vi "[RT] eHS Main.vi"() -> ()   [LabVIEW 2017]
uses:
  <vilib>/userdefined/High Color/nirio_resource_hc.ctl
  <vilib>/NI/cRIO Wfm/ChannelConfig.ctl
  <vilib>/OPAL-RT/Utilities Toolkit/Mapping/Input Mapping/Common/Controls/Input Mapping Parameters.ctl
  <vilib>/OPAL-RT/Utilities Toolkit/Mapping/Input Mapping/Common/Controls/Input Source Types.ctl
  <vilib>/OPAL-RT/Utilities Toolkit/Mapping/Switch Mapping/Common/Controls/Switch Mapping Parameters.ctl
  <vilib>/OPAL-RT/Utilities Toolkit/Mapping/Switch Mapping/Common/Controls/Switch Source Types.ctl
  <vilib>/OPAL-RT/Analog I-O Mapping & Conditioning Toolkit/AOMC/Common/Public/Controls/AOMC Configuration Parameters.ctl
  <vilib>/OPAL-RT/Analog I-O Mapping & Conditioning Toolkit/AOMC/Common/Public/Controls/AO Mapping Parameters.ctl
  <vilib>/OPAL-RT/Analog I-O Mapping & Conditioning Toolkit/AOMC/Common/Public/Controls/Source Type.ctl
  <vilib>/OPAL-RT/Analog I-O Mapping & Conditioning Toolkit/AOMC/Common/Public/Controls/AO Conditioning Parameters.ctl
  <vilib>/OPAL-RT/eHS Toolkit/eHS Host/Controls/eHS Core Index.ctl
  <vilib>/OPAL-RT/FPGA Signal Generation Toolkit/Sinewave Generation/Host/Public/Controls/Phase Offset Mode.ctl
  <vilib>/OPAL-RT/FPGA Signal Generation Toolkit/Sinewave Generation/Host/Public/Controls/Sinewave FPGA Clock Rate.ctl
  <vilib>/OPAL-RT/FPGA Signal Generation Toolkit/Sinewave Generation/Host/Public/Controls/Sinewave RT Configuration Parameters.ctl
  <vilib>/OPAL-RT/FPGA Signal Generation Toolkit/Sinewave Generation/Host/Public/Controls/Sinewave Generator Action.ctl
  <vilib>/OPAL-RT/eHS Toolkit/eHS Host/SubVIs/eHS Core/eHSx64 Initialize Solver Core.vi
  <vilib>/OPAL-RT/Analog I-O Mapping & Conditioning Toolkit/AOMC/Host/Private/Pack & Send AOMC Configuration Setting.vi
  <vilib>/Utility/error.llb/Error Cluster From Error Code.vi
  <vilib>/rvi/errors/niLvFpgaAdjustHostInterfaceError.vi
  <vilib>/NI/cRIO Wfm/AcqRead(Wfm).vi
  <vilib>/FPGAPlugInAG/Dynamic/niLvFpga_Abort_Dynamic.vi
  <vilib>/FPGAPlugInAG/Dynamic/niLvFpga_Close_Dynamic.vi
  <vilib>/rvi/interface/nirviReadWriteControl/nirviReadWriteControl.xnode
  Controls/eHS FPGA Ref.ctl
  <vilib>/rvi/interface/nirviMethod/nirviMethod.xnode
  <vilib>/rvi/interface/nirviCloseFPGA/nirviCloseFPGA.xnode
  <vilib>/NI/cRIO Wfm/cRIO Wfm.lvlib
  <vilib>/OPAL-RT/eHS Toolkit/eHS Host/eHS - Host.lvlib
  <vilib>/OPAL-RT/Analog I-O Mapping & Conditioning Toolkit/AOMC/Host/AO Mapping & Conditioning - Host.lvlib
  <vilib>/OPAL-RT/FPGA Signal Generation Toolkit/Sinewave Generation/Host/Sinewave Generation - Host.lvlib
  <vilib>/rvi/interface/Simulation/niFpgaSimulationCallBeginRW.vi
  NiFpgaLv.dll
  <vilib>/OPAL-RT/Utilities Toolkit/Mapping/Input Mapping/Common/Input Mapping - Common.lvlib
  <vilib>/OPAL-RT/Utilities Toolkit/Mapping/Switch Mapping/Common/Switch Mapping - Common.lvlib
  <vilib>/OPAL-RT/Analog I-O Mapping & Conditioning Toolkit/AOMC/Common/AO Mapping & Conditioning - Common.lvlib
panel:
  in  "STOP":bool
  in  "eHS+PMSM Tab":T1(tab)=enum."Control & Monitor"
  in  "Resource name":T2="RIO0" caption="RIO Device"
  in  "Waveform Channel Info":T3=[{"Channel Name"="U01", "Sensitivity mV_EU"=1000.0, "EU"="V", "dB Ref EU"=1.0}, {"Channel Name"="U02", "Sensitivity mV_EU"=1000.0, "EU"="V", "dB Ref EU"=1.0}, {"Channel Name"="U03", "Sensitivity mV_EU"=1000.0, "EU"="V", "dB Ref EU"=1.0}, {"Channel Name"="U04", "Sensitivity mV_EU"=1000.0, "EU"="V", "dB Ref EU"=1.0}, {"Channel Name"="U05", "Sensitivity mV_EU"=1000.0, "EU"="V", "dB Ref EU"=1.0}, {"Channel Name"="U06", "Sensitivity mV_EU"=1000.0, "EU"="V", "dB Ref EU"=1.0}, {"Channel Name"="U07", "Sensitivity mV_EU"=1000.0, "EU"="V", "dB Ref EU"=1.0}, {"Channel Name"="U08", "Sensitivity mV_EU"=1000.0, "EU"="V", "dB Ref EU"=1.0}, {"Channel Name"="U09", "Sensitivity mV_EU"=1000.0, "EU"="V", "dB Ref EU"=1.0}, {"Channel Name"="U10", "Sensitivity mV_EU"=1000.0, "EU"="V", "dB Ref EU"=1.0}, {"Channel Name"="U11", "Sensitivity mV_EU"=1000.0, "EU"="V", "dB Ref EU"=1.0}, {"Channel Name"="U12", "Sensitivity mV_EU"=1000.0, "EU"="V", "dB Ref EU"=1.0}, {"Channel Name"="U13", "Sensitivity mV_EU"=1000.0, "EU"="V", "dB Ref EU"=1.0}, {"Channel Name"="U14", "Sensitivity mV_EU"=1000.0, "EU"="V", "dB Ref EU"=1.0}, {"Channel Name"="U15", "Sensitivity mV_EU"=1000.0, "EU"="V", "dB Ref EU"=1.0}, {"Channel Name"="U16", "Sensitivity mV_EU"=1000.0, "EU"="V", "dB Ref EU"=1.0}, {"Channel Name"="U17", "Sensitivity mV_EU"=1000.0, "EU"="V", "dB Ref EU"=1.0}, {"Channel Name"="U18", "Sensitivity mV_EU"=1000.0, "EU"="V", "dB Ref EU"=1.0}, {"Channel Name"="U19", "Sensitivity mV_EU"=1000.0, "EU"="V", "dB Ref EU"=1.0}, {"Channel Name"="U20", "Sensitivity mV_EU"=1000.0, "EU"="V", "dB Ref EU"=1.0}, {"Channel Name"="U21", "Sensitivity mV_EU"=1000.0, "EU"="V", "dB Ref EU"=1.0}, {"Channel Name"="U22", "Sensitivity mV_EU"=1000.0, "EU"="V", "dB Ref EU"=1.0}, {"Channel Name"="U23", "Sensitivity mV_EU"=1000.0, "EU"="V", "dB Ref EU"=1.0}, {"Channel Name"="U24", "Sensitivity mV_EU"=1000.0, "EU"="V", "dB Ref EU"=1.0}, {"Channel Name"="U25", "Sensitivity mV_EU"=1000.0, "EU"="V", "dB Ref EU"=1.0}, {"Channel Name"="U26", "Sensitivity mV_EU"=1000.0, "EU"="V", "dB Ref EU"=1.0}, {"Channel Name"="U27", "Sensitivity mV_EU"=1000.0, "EU"="V", "dB Ref EU"=1.0}, {"Channel Name"="U28", "Sensitivity mV_EU"=1000.0, "EU"="V", "dB Ref EU"=1.0}, {"Channel Name"="U29", "Sensitivity mV_EU"=1000.0, "EU"="V", "dB Ref EU"=1.0}, {"Channel Name"="U30", "Sensitivity mV_EU"=1000.0, "EU"="V", "dB Ref EU"=1.0}, {"Channel Name"="U31", "Sensitivity mV_EU"=1000.0, "EU"="V", "dB Ref EU"=1.0}, {"Channel Name"="U32", "Sensitivity mV_EU"=1000.0, "EU"="V", "dB Ref EU"=1.0}] {"dB Ref EU" format="%#.2p"; "Sensitivity mV_EU" format="%.2f"}
  in  "Waveform Buffer Size":i32=100000
  in  "Waveform Sample Rate":u32=88888
  in  "eHS Input Mapping Keys":T4[](array[typedef])=[{"Source Index"=0, "Input Source Types"=enum."Group B"}, {"Source Index"=1, "Input Source Types"=enum."Group B"}, {"Source Index"=2, "Input Source Types"=enum."Group B"}, {"Source Index"=3, "Input Source Types"=enum."Group B"}, {"Source Index"=4, "Input Source Types"=enum."Group B"}, {"Source Index"=5, "Input Source Types"=enum."Group B"}, {"Source Index"=0, "Input Source Types"=enum."Group A"}]
  in  "eHS Switch Mapping Keys":T6[](array[typedef])=[{"Switch Source Types"=enum."Group D", "Source Index"=0, "Invert?"=FALSE}, {"Switch Source Types"=enum."Group D", "Source Index"=1, "Invert?"=FALSE}, {"Switch Source Types"=enum."Group D", "Source Index"=2, "Invert?"=FALSE}, {"Switch Source Types"=enum."Group D", "Source Index"=3, "Invert?"=FALSE}, {"Switch Source Types"=enum."Group D", "Source Index"=4, "Invert?"=FALSE}, {"Switch Source Types"=enum."Group D", "Source Index"=5, "Invert?"=FALSE}, {"Switch Source Types"=enum."Group D", "Source Index"=6, "Invert?"=FALSE}, {"Switch Source Types"=enum."Group D", "Source Index"=7, "Invert?"=FALSE}, {"Switch Source Types"=enum."Group D", "Source Index"=8, "Invert?"=FALSE}, {"Switch Source Types"=enum."Group D", "Source Index"=9, "Invert?"=FALSE}, {"Switch Source Types"=enum."Group D", "Source Index"=10, "Invert?"=TRUE}, {"Switch Source Types"=enum."Group D", "Source Index"=11, "Invert?"=FALSE}]
  in  "AOMC Configuration Parameters":T8[](array[typedef])=[{"AO Mapping Parameters"={"AO Channel Index"=0, "Source"=enum."Group A", "Source Index"=8}, "AO Conditioning Parameters"={"Scaling Factor"=0.5, "Offset Factor"=0.0, "Minumum Saturation"=-10.0, "Maximum Saturation"=10.0}}, {"AO Mapping Parameters"={"AO Channel Index"=1, "Source"=enum."Group A", "Source Index"=9}, "AO Conditioning Parameters"={"Scaling Factor"=0.5, "Offset Factor"=0.0, "Minumum Saturation"=-10.0, "Maximum Saturation"=10.0}}, {"AO Mapping Parameters"={"AO Channel Index"=2, "Source"=enum."Not Connected", "Source Index"=0}, "AO Conditioning Parameters"={"Scaling Factor"=0.0, "Offset Factor"=0.0, "Minumum Saturation"=-10.0, "Maximum Saturation"=10.0}}, {"AO Mapping Parameters"={"AO Channel Index"=3, "Source"=enum."Not Connected", "Source Index"=0}, "AO Conditioning Parameters"={"Scaling Factor"=0.0, "Offset Factor"=0.0, "Minumum Saturation"=-10.0, "Maximum Saturation"=10.0}}, {"AO Mapping Parameters"={"AO Channel Index"=4, "Source"=enum."Group A", "Source Index"=6}, "AO Conditioning Parameters"={"Scaling Factor"=0.014793, "Offset Factor"=0.0, "Minumum Saturation"=-10.0, "Maximum Saturation"=10.0}}, {"AO Mapping Parameters"={"AO Channel Index"=5, "Source"=enum."Not Connected", "Source Index"=0}, "AO Conditioning Parameters"={"Scaling Factor"=0.0, "Offset Factor"=0.0, "Minumum Saturation"=0.0, "Maximum Saturation"=0.0}}, {"AO Mapping Parameters"={"AO Channel Index"=6, "Source"=enum."Not Connected", "Source Index"=0}, "AO Conditioning Parameters"={"Scaling Factor"=0.0, "Offset Factor"=0.0, "Minumum Saturation"=0.0, "Maximum Saturation"=0.0}}, {"AO Mapping Parameters"={"AO Channel Index"=7, "Source"=enum."Not Connected", "Source Index"=0}, "AO Conditioning Parameters"={"Scaling Factor"=0.0, "Offset Factor"=0.0, "Minumum Saturation"=0.0, "Maximum Saturation"=0.0}}, {"AO Mapping Parameters"={"AO Channel Index"=8, "Source"=enum."Group A", "Source Index"=3}, "AO Conditioning Parameters"={"Scaling Factor"=0.5, "Offset Factor"=0.0, "Minumum Saturation"=-10.0, "Maximum Saturation"=10.0}}, {"AO Mapping Parameters"={"AO Channel Index"=9, "Source"=enum."Group A", "Source Index"=4}, "AO Conditioning Parameters"={"Scaling Factor"=0.5, "Offset Factor"=0.0, "Minumum Saturation"=-10.0, "Maximum Saturation"=10.0}}, {"AO Mapping Parameters"={"AO Channel Index"=10, "Source"=enum."Group A", "Source Index"=5}, "AO Conditioning Parameters"={"Scaling Factor"=0.5, "Offset Factor"=0.0, "Minumum Saturation"=-10.0, "Maximum Saturation"=10.0}}, {"AO Mapping Parameters"={"AO Channel Index"=11, "Source"=enum."Group A", "Source Index"=7}, "AO Conditioning Parameters"={"Scaling Factor"=0.1, "Offset Factor"=0.0, "Minumum Saturation"=-10.0, "Maximum Saturation"=10.0}}, {"AO Mapping Parameters"={"AO Channel Index"=12, "Source"=enum."Group A", "Source Index"=0}, "AO Conditioning Parameters"={"Scaling Factor"=0.04714, "Offset Factor"=0.0, "Minumum Saturation"=-10.0, "Maximum Saturation"=10.0}}, {"AO Mapping Parameters"={"AO Channel Index"=13, "Source"=enum."Group A", "Source Index"=1}, "AO Conditioning Parameters"={"Scaling Factor"=0.04714, "Offset Factor"=0.0, "Minumum Saturation"=-10.0, "Maximum Saturation"=10.0}}, {"AO Mapping Parameters"={"AO Channel Index"=14, "Source"=enum."Group A", "Source Index"=2}, "AO Conditioning Parameters"={"Scaling Factor"=0.04714, "Offset Factor"=0.0, "Minumum Saturation"=-10.0, "Maximum Saturation"=10.0}}, {"AO Mapping Parameters"={"AO Channel Index"=15, "Source"=enum."Group A", "Source Index"=10}, "AO Conditioning Parameters"={"Scaling Factor"=0.014793, "Offset Factor"=0.0, "Minumum Saturation"=-10.0, "Maximum Saturation"=10.0}}]
  out "eHS Outputs":waveform(sgl)[](graph)=[{"t0"=timestamp(3605532672.448228 s since 1904-01-01), "dt"=1.1249999999999999e-05, "Y"=array[10000 elements], "attributes"=variant("NI_ChannelName"=variant(string "U04"), "NI_UnitDescription"=variant(string "V"), "NI_dBReference"=variant(dbl 1.0))}, {"t0"=timestamp(3605532672.448228 s since 1904-01-01), "dt"=1.1249999999999999e-05, "Y"=array[10000 elements], "attributes"=variant("NI_ChannelName"=variant(string "U05"), "NI_UnitDescription"=variant(string "V"), "NI_dBReference"=variant(dbl 1.0))}, {"t0"=timestamp(3605532672.448228 s since 1904-01-01), "dt"=1.1249999999999999e-05, "Y"=array[10000 elements], "attributes"=variant("NI_ChannelName"=variant(string "U06"), "NI_UnitDescription"=variant(string "V"), "NI_dBReference"=variant(dbl 1.0))}]
  in  "eHS Constant Inputs":sgl[](array[numeric])=[12.6, 0.0, 0.0, 0.0, 0.0, 0.0, 0.0, 0.0, 0.0, 0.0, 0.0, 0.0, 0.0, 0.0, 0.0, 0.0, 0.0, 0.0, 0.0, 0.0, 0.0, 0.0, 0.0, 0.0, 0.0, 0.0, 0.0, 0.0, 0.0, 0.0, 0.0, 0.0]
  in  "eHS SW Constants":bool[](array[boolean])=[FALSE, FALSE, FALSE, FALSE, FALSE, FALSE, FALSE, FALSE, FALSE, FALSE, FALSE, FALSE, FALSE, FALSE, FALSE, FALSE, FALSE, FALSE, FALSE, FALSE, FALSE, FALSE, FALSE, FALSE, FALSE, FALSE, FALSE, FALSE, FALSE, FALSE, FALSE, FALSE, FALSE, FALSE, FALSE, FALSE, FALSE, FALSE, FALSE, FALSE, FALSE, FALSE, FALSE, FALSE, FALSE, FALSE, FALSE, FALSE, FALSE, FALSE, FALSE, FALSE, FALSE, FALSE, FALSE, FALSE, FALSE, FALSE, FALSE, FALSE, FALSE, FALSE, FALSE, FALSE, FALSE, FALSE, FALSE, FALSE, FALSE, FALSE, FALSE, FALSE]
  in  "Waveform Selection":T12={"Boolean"=FALSE, "Boolean 2"=FALSE, "Boolean 3"=FALSE, "Boolean 4"=TRUE, "Boolean 5"=TRUE, "Boolean 6"=TRUE, "Boolean 7"=FALSE, "Boolean 8"=FALSE, "Boolean 9"=FALSE, "Boolean 10"=FALSE, "Boolean 11"=FALSE, "Boolean 12"=FALSE, "Boolean 13"=FALSE, "Boolean 14"=FALSE, "Boolean 15"=FALSE, "Boolean 16"=FALSE, "Boolean 17"=FALSE, "Boolean 18"=FALSE, "Boolean 19"=FALSE, "Boolean 20"=FALSE, "Boolean 21"=FALSE, "Boolean 22"=FALSE, "Boolean 23"=FALSE, "Boolean 24"=FALSE, "Boolean 25"=FALSE, "Boolean 26"=FALSE, "Boolean 27"=FALSE, "Boolean 28"=FALSE, "Boolean 29"=FALSE, "Boolean 30"=FALSE, "Boolean 31"=FALSE, "Boolean 32"=FALSE}
  out "Mapped & Conditioned Data_Debug":fxp<+/-,20,5>[](array[numeric])=[10.0, 10.0, 0.0, 0.0, 3.26995849609375, 0.0, 0.0, 0.0, 10.0, -8.520599365234375, 10.0, 3.556671142578125, 7.373077392578125, -3.07159423828125, -5.40924072265625, 3.2708740234375, 0.0, 0.0, 0.0, 0.0, 0.0, 0.0, 0.0, 0.0, 0.0, 0.0, 0.0, 0.0, 0.0, 0.0, 0.0, 0.0] format="%.17g"
  out "Conditioned AI Data_Debug":sgl[](array[numeric])
  # "Hardware Setup"
  # "RIO Waveform Settings"
  # "eHS U #"
  # "eHS SW #"
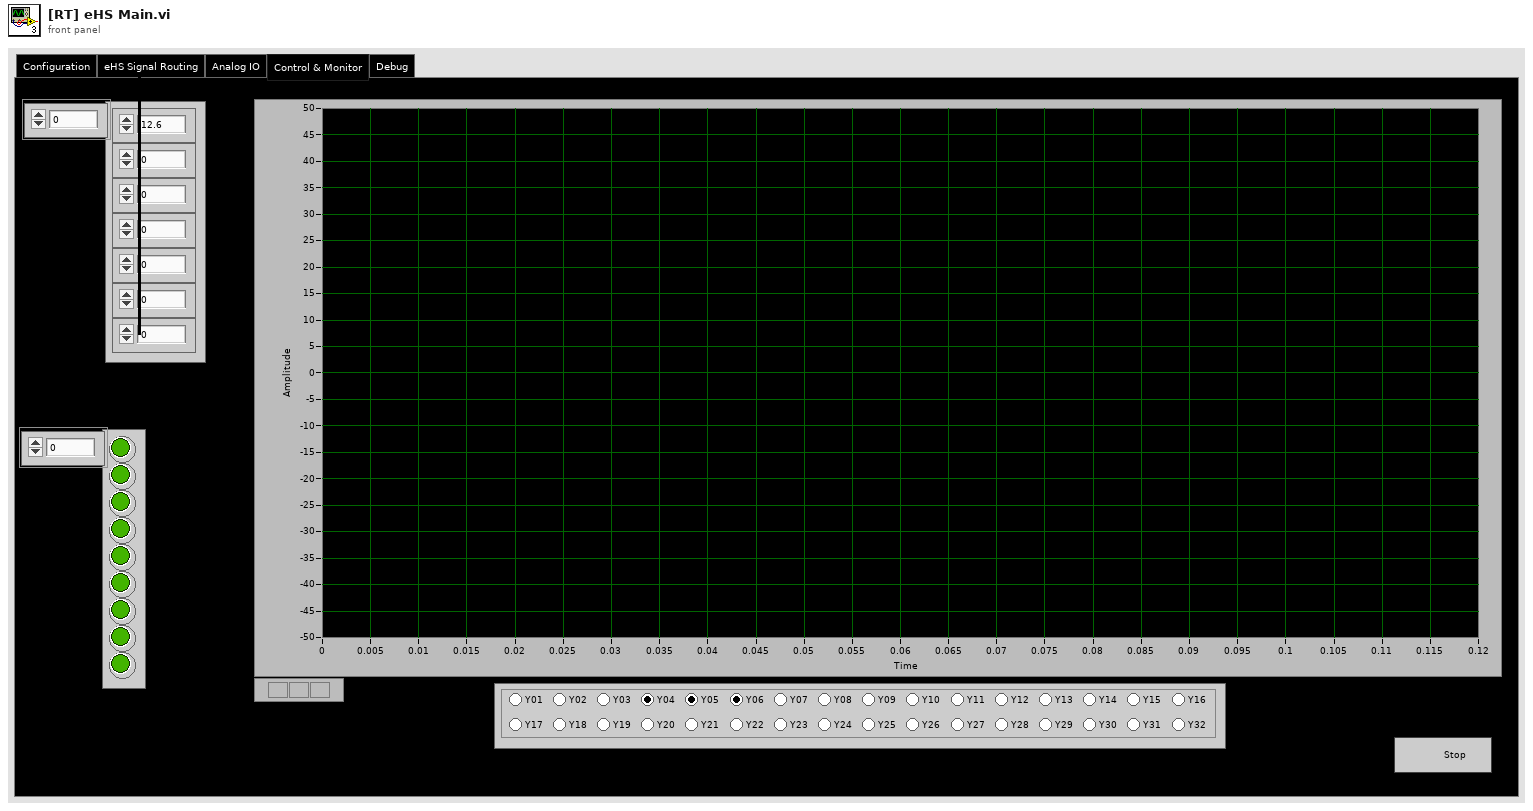
[diagram p1: front panel]
types:
  T1 = enum32{"Configuration", "eHS Signal Routing", "Analog IO", "Control & Monitor", "Debug"}
  T2 = typedef "nirio_resource_hc.ctl" = tag
  T3 = typedef "cRIO Wfm.lvlib/ChannelConfig.ctl" = cluster{"Channel Name":string, "Sensitivity mV_EU":dbl, "EU":string, "dB Ref EU":dbl}[]
  T4 = typedef "Input Mapping - Common.lvlib/Input Mapping Parameters.ctl" = cluster{"Source Index":u8, "Input Source Types":T5}
  T5 = typedef "Input Mapping - Common.lvlib/Input Source Types.ctl" = enum16{"Not Connected", "Group A", "Group B", "Group C", "Group D"}
  T6 = typedef "Switch Mapping - Common.lvlib/Switch Mapping Parameters.ctl" = cluster{"Switch Source Types":T7, "Source Index":u8, "Invert?":bool}
  T7 = typedef "Switch Mapping - Common.lvlib/Switch Source Types.ctl" = enum16{"Not Connected", "Group A", "Group B", "Group C", "Group D", "Group E"}
  T8 = typedef "AO Mapping & Conditioning - Common.lvlib/AOMC Configuration Parameters.ctl" = cluster{"AO Mapping Parameters":T9, "AO Conditioning Parameters":T11}
  T9 = typedef "AO Mapping & Conditioning - Common.lvlib/AO Mapping Parameters.ctl" = cluster{"AO Channel Index":u8, "Source":T10, "Source Index":u8}
  T10 = typedef "AO Mapping & Conditioning - Common.lvlib/Source Type.ctl" = enum16{"Not Connected", "Group A", "Group B"}
  T11 = typedef "AO Mapping & Conditioning - Common.lvlib/AO Conditioning Parameters.ctl" = cluster{"Scaling Factor":sgl, "Offset Factor":sgl, "Minumum Saturation":sgl, "Maximum Saturation":sgl}
  T12 = cluster{"Boolean":bool, "Boolean 2":bool, "Boolean 3":bool, "Boolean 4":bool, "Boolean 5":bool, "Boolean 6":bool, "Boolean 7":bool, "Boolean 8":bool, "Boolean 9":bool, "Boolean 10":bool, "Boolean 11":bool, "Boolean 12":bool, "Boolean 13":bool, "Boolean 14":bool, "Boolean 15":bool, "Boolean 16":bool, "Boolean 17":bool, "Boolean 18":bool, "Boolean 19":bool, "Boolean 20":bool, "Boolean 21":bool, "Boolean 22":bool, "Boolean 23":bool, "Boolean 24":bool, "Boolean 25":bool, "Boolean 26":bool, "Boolean 27":bool, "Boolean 28":bool, "Boolean 29":bool, "Boolean 30":bool, "Boolean 31":bool, "Boolean 32":bool}
  T13 = typedef "Sinewave Generation - Host.lvlib/Sinewave Generator Action.ctl" = enum16{"Do Nothing", "Stop", "Re-Start"}
  T14 = typedef "Sinewave Generation - Host.lvlib/Sinewave RT Configuration Parameters.ctl" = cluster{"Frequency Engine Index":u8, "Phase Offset (Deg\\Rad)":dbl, "Amplitude":dbl, "Offset":dbl}
  T15 = typedef "Sinewave Generation - Host.lvlib/Sinewave FPGA Clock Rate.ctl" = enum16{"50MHz", "100MHz"}
  T16 = typedef "Sinewave Generation - Host.lvlib/Phase Offset Mode.ctl" = enum16{"Degrees", "Radians"}
  T17 = typedef "OPAL-RT eHS.lvlib/eHS - Host.lvlib/eHS Core Index.ctl" = enum16{"Core 1", "Core 2", "Core 3", "Core 4", "Core 5", "Core 6", "Core 7", "Core 8", "Core 9", "Core 10"}
  T18 = typedef "eHS FPGA Ref.ctl" = refnum<k20>
  T19 = typedef "cRIO Wfm.lvlib/SamplingInfo.ctl" = cluster{"Number of Channels":i32, "Actual Samp Rate":dbl, "Chan Name Array":string[], "EU Chan Array":string[], "dB Ref Chan Array":dbl[]}
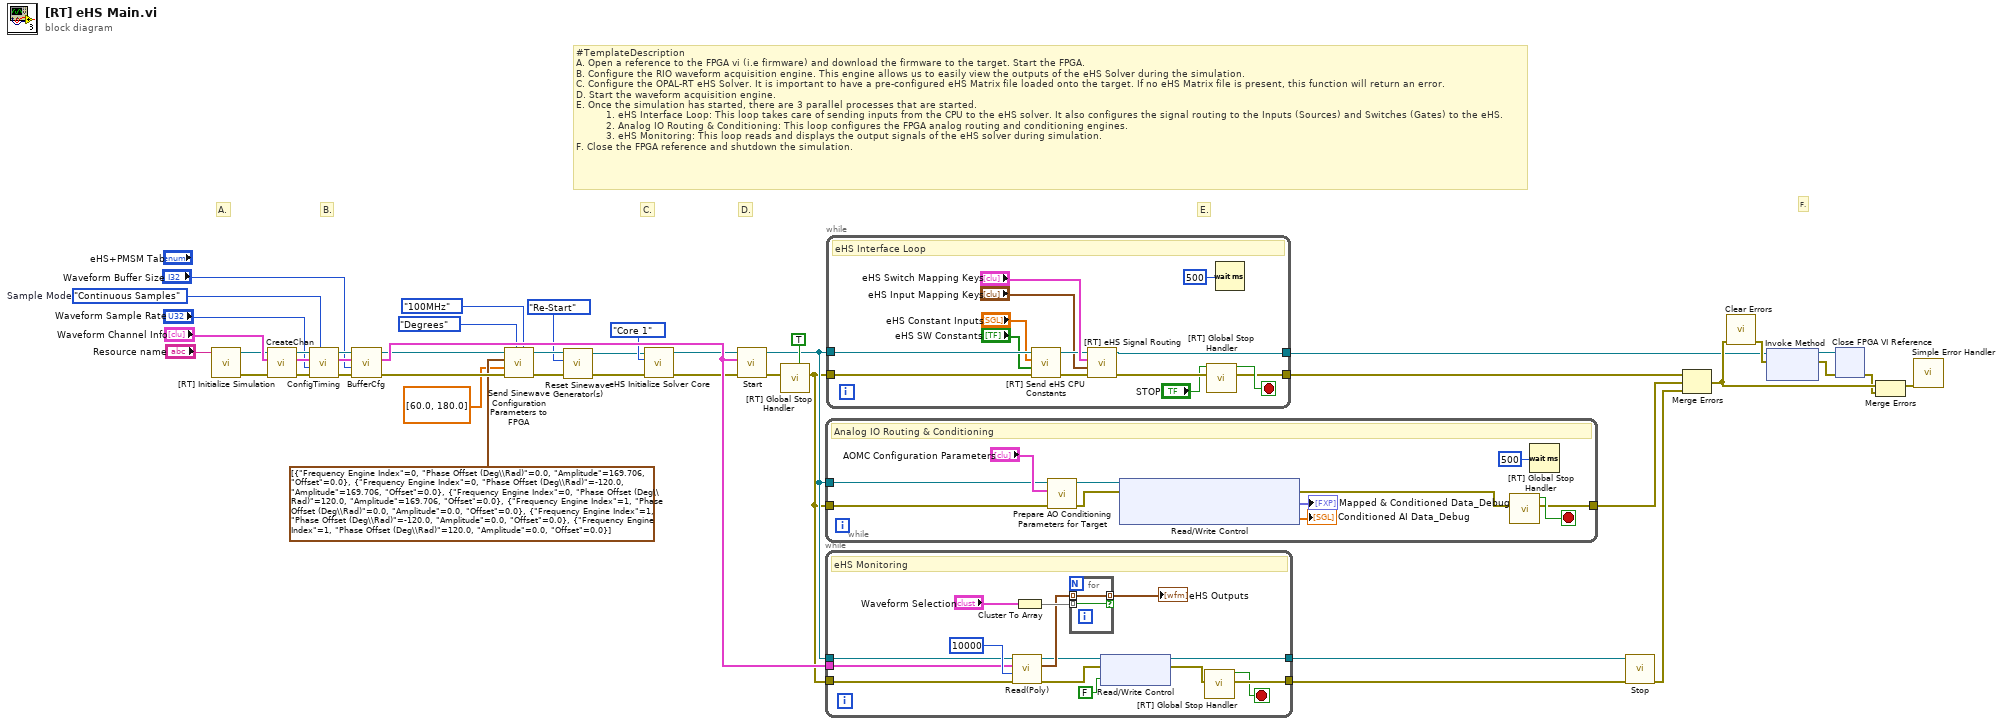
[diagram p0: block diagram]
diagram:
  w37 = enum16{"Finite Samples", "Continuous Samples"}."Continuous Samples"  # Sample Mode
  # "#TemplateDescription\nA.\tOpen a reference to the FPGA vi (i.e firmware) and download the firmware to the target. Start the FPGA.\nB.\tConfigure the RIO waveform acquisition engine. This engine allows us to easily view the outputs of the eHS Solver during the simulation.\nC.\tConfigure the OPAL-RT eHS Solver. It is important to have a pre-configured eHS Matrix file loaded onto the target. If no eHS Matrix file is present, this function will return an error.\nD.\tStart the waveform acquisition engine.\nE.\tOnce the simulation has started, there are 3 parallel processes that are started.        \n          1.\teHS Interface Loop: This loop takes care of sending inputs from the CPU to the eHS solver. It also configures the signal routing to the Inputs (Sources) and Switches (Gates) to the eHS. \n          2.\tAnalog IO Routing & Conditioning: This loop configures the FPGA analog routing and conditioning engines. \n          3.\teHS Monitoring: This loop reads and displays the output signals of the eHS solver during simulation. \nF.\tClose the FPGA reference and shutdown the simulation."
  # "F."
  # "E."
  # "D."
  # "C."
  # "B."
  # "A."
  n1 = call "[RT] Initialize Simulation.vi"("Resource name"="Resource name") -> ("Error out"=w18:errorcluster, "FPGA VI reference"=w19:T18)  [unwired: 9 in]
  n2 = call <vilib>:"CreateChan.vi"("error in"=w18, "Channel Info"="Waveform Channel Info", "Dynamic FPGA Ref"=w19) -> ("error out"=w43:errorcluster, "Sampling Info"=w40:T19, "Dynamic FPGA Ref Out"=w44:T18)  [unwired: 6 in]
  n3 = call <vilib>:"ConfigTiming.vi"("Sample Mode"=w37, "error in"=w43, "Sample Rate"="Waveform Sample Rate", "Sampling Info In"=w40, "Dynamic FPGA Ref"=w44) -> ("error out"=w42:errorcluster, "Sampling Info Out"=w39:T19, "Dynamic FPGA Ref Out"=w41:T18)  [unwired: 3 in, 1 out]
  n4 = call <vilib>:"BufferCfg.vi"("error in"=w42, "Buffer Size [Samps per Chan]"="Waveform Buffer Size", "Sampling Info In"=w39, "Dynamic FPGA Ref"=w41) -> ("error out"=w10:errorcluster, "Sampling Info Out"=w34:T19, "Dynamic FPGA Ref Out"=w11:T18)  [unwired: 4 in, 1 out]
  n5 = call <vilib>:"Send Sinewave Configuration Parameters to FPGA.vi"("Sinewave FPGA Clock Rate"=Sinewave_FPGA_Clock_Rate."100MHz", "Phase Offset Mode"=Phase_Offset_Mode."Degrees", "Error In"=w10, "Frequency Engine Configuration"=dbl[] [60.0, 180.0] ("Sinewave RT Frequency Engine Configuration Parameters"), "Sinewave Configuration Parameters"=T14[] [{"Frequency Engine Index"=0, "Phase Offset (Deg\\Rad)"=0.0, "Amplitude"=169.706, "Offset"=0.0}, {"Frequency Engine Index"=0, "Phase Offset (Deg\\Rad)"=-120.0, "Amplitude"=169.706, "Offset"=0.0}, {"Frequency Engine Index"=0, "Phase Offset (Deg\\Rad)"=120.0, "Amplitude"=169.706, "Offset"=0.0}, {"Frequency Engine Index"=1, "Phase Offset (Deg\\Rad)"=0.0, "Amplitude"=0.0, "Offset"=0.0}, {"Frequency Engine Index"=1, "Phase Offset (Deg\\Rad)"=-120.0, "Amplitude"=0.0, "Offset"=0.0}, {"Frequency Engine Index"=1, "Phase Offset (Deg\\Rad)"=120.0, "Amplitude"=0.0, "Offset"=0.0}], "Sinewave FPGA Reference In"=w11) -> ("Error Out"=w4:errorcluster, "Sinewave FPGA Reference Out"=w5:T18)  [unwired: 4 in]
  n6 = call <vilib>:"Reset Sinewave Generator(s).vi"("Error In"=w4, "Sinewave Generator Action"=Sinewave_Generator_Action."Re-Start", "Sinewave FPGA Reference In"=w5) -> ("Error Out"=w2:errorcluster, "Sinewave FPGA Reference Out"=w3:T18)  [unwired: 7 in]
  n7 = call-poly <vilib>:"eHS Initialize Solver Core.vi"("Error In"=w2, "eHS Core ID"=eHS_Core_Index."Core 1", "eHS FPGA VI Reference In"=w3) -> ("Error Out"=w22:errorcluster, "eHS FPGA VI Reference Out"=w17:T18)  [unwired: 7 in]
  n8 = call <vilib>:"Start.vi"("error in"=w22, "Sampling Info In"=w34, "Dynamic FPGA Ref"=w17) -> ("error out"=w33:errorcluster, "Dynamic FPGA Ref Out"=w13:T18)  [unwired: 6 in, 1 out]
  n9 = call "[RT] Global Stop Handler.vi"("Reset?"=TRUE, "Error In"=w33) -> ("Error Out"=w12:errorcluster)  [unwired: 6 in, 1 out]
  n10 = while {
    tunnel: w13 -> [w52]
    tunnel: w12 -> [w51]
    tunnel: [w53] -> w14
    stop <- w54 stop-if-true
    # "Analog IO Routing & Conditioning"
    n11 = call-poly <vilib>:"Prepare AO Conditioning Parameters for Target.vi"("Error In"=w51, "AOMC Configuration Parameters"="AOMC Configuration Parameters", "AO FPGA VI Reference In"=w52) -> ("Error Out"=w48:errorcluster, "AO FPGA VI Reference Out"=w49:T18)  [unwired: 7 in]
    n12 = xnode "Read/Write Control"("FPGA VI Reference In"=w49, "error in"=w48) -> ("error out"=w47:errorcluster, "Mapped & Conditioned Data_Debug"=→"Mapped & Conditioned Data_Debug":fxp<+/-,20,5>[], "Conditioned AI Data_Debug"=→"Conditioned AI Data_Debug":sgl[])  [unwired: 1 out]
    n13 = call "[RT] Global Stop Handler.vi"("Error In"=w47) -> ("Error Out"=w53:errorcluster, "Stop?"=w54:bool)  [unwired: 7 in]
    n14 = Wait (ms)(milliseconds to wait=u32 500) -> ()  [unwired: 1 out]
  }
  n15 = while {
    tunnel: w34 -> [w69]
    tunnel: [w68] -> w30
    tunnel: w12 -> [w66]
    tunnel: w13 -> [w65]
    tunnel: [w58] -> w29
    stop <- w67 stop-if-true
    # "eHS Monitoring"
    n16 = call-poly <vilib>:"Read(Poly).vi"("error in"=w66, "Samps Read per Chan"=10000, "Sampling Info"=w69, "Dynamic FPGA Ref"=w65) -> ("error out"=w59:errorcluster, "Wfm Data"=w62:waveform(sgl)[], "Dynamic FPGA Ref Out"=w60:T18)  [unwired: 4 in, 1 out]
    n17 = Cluster To Array(cluster="Waveform Selection") -> (array=w64:bool[])
    n18 = for {
      tunnel: [w72] -> w61 mode=indexing if=w71
      tunnel: w62 -> [w72] mode=indexing
      tunnel: w64 -> [w71] mode=indexing
    }
    "eHS Outputs" <- w61
    n19 = xnode "Read/Write Control"("FPGA VI Reference In"=w60, "error in"=w59, "View SPWM"=FALSE) -> ("FPGA VI Reference Out"=w58:T18, "error out"=w57:errorcluster)
    n20 = call "[RT] Global Stop Handler.vi"("Error In"=w57) -> ("Error Out"=w68:errorcluster, "Stop?"=w67:bool)  [unwired: 7 in]
  }
  n21 = while {
    tunnel: w12 -> [w79]
    tunnel: w13 -> [w81]
    tunnel: [w85] -> w15
    tunnel: [w74] -> w16
    stop <- w86 stop-if-true
    # "eHS Interface Loop"
    n22 = call "[RT] Send eHS CPU Constants.vi"("Error In"=w79, "eHS SW Constants"="eHS SW Constants", "eHS Constant Inputs"="eHS Constant Inputs", "FPGA Reference In"=w81) -> ("Error Out"=w78:errorcluster, "FPGA Reference Out"=w80:T18)  [unwired: 6 in]
    n23 = call "[RT] eHS Signal Routing.vi"("Error In"=w78, "eHS Input Mapping Keys"="eHS Input Mapping Keys", "eHS Switch Mapping Keys"="eHS Switch Mapping Keys", "FPGA VI Reference In"=w80) -> ("Error Out"=w82:errorcluster, "FPGA VI Reference Out"=w74:T18)  [unwired: 6 in]
    n24 = call "[RT] Global Stop Handler.vi"("Error In"=w82, "Initiate Stop?"="STOP") -> ("Error Out"=w85:errorcluster, "Stop?"=w86:bool)  [unwired: 6 in]
    n25 = Wait (ms)(milliseconds to wait=u32 500) -> ()  [unwired: 1 out]
  }
  n26 = call <vilib>:"Stop.vi"("error in"=w30, "Dynamic FPGA Ref"=w29) -> ("error out"=w31:errorcluster)  [unwired: 8 in, 1 out]
  n27 = Merge Errors(w15, w14, w31) -> (w24:errorcluster)
  n28 = call <vilib>:"Clear Errors.vi"("error in (no error)"=w24) -> ("error out"=w26:errorcluster)  [unwired: 5 in, 1 out]
  n29 = xnode "Invoke Method"("FPGA VI Reference In"=w16, "error in"=w26) -> ("FPGA VI Reference Out"=w28:T18, "error out"=w27:errorcluster)
  n30 = xnode "Close FPGA VI Reference"("FPGA VI Reference In"=w28, "error in"=w27) -> ("error out"=w23:errorcluster)
  n31 = Merge Errors(w24, w23) -> (w25:errorcluster)
  n32 = call <vilib>:"Simple Error Handler.vi"("error in (no error)"=w25) -> ()  [unwired: 4 in, 5 out]
